vi "find_PipObject_by_InnerSwitchName.vi"(10 "inner switch name":string, 11 "PipObj Array in":refnum<class "Pipette.lvclass">[](array[class])) -> (0 "index of Object in Array":i32, 1 "found?":bool, 2 "found PipObj out":refnum<class "Pipette.lvclass">, 3 "PipObj Array out":refnum<class "Pipette.lvclass">[](array[class]))   [LabVIEW 2017]
doc: "Find the correct PipetteObject by the Name of the Inner Switch"
uses:
  Classes/Pipette/Pipette.lvclass
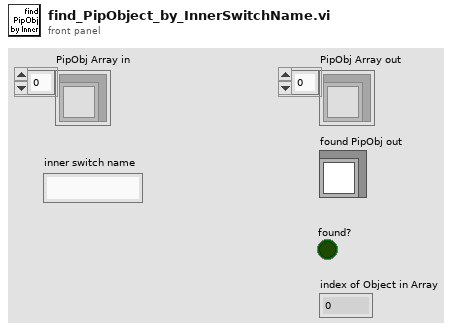
[diagram p1: front panel]
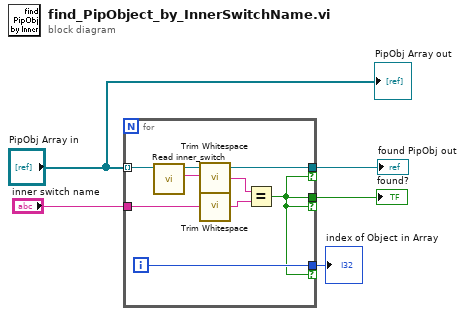
[diagram p0: block diagram]
diagram:
  n1 = for {
    tunnel: "inner switch name" -> [w13]
    tunnel: [w10] -> w4 if=w6
    tunnel: "PipObj Array in" -> [w8] mode=indexing
    tunnel: [w6] -> w3 if=w6
    tunnel: [w7] -> w1 if=w6
    i -> [w7]
    n2 = call-dynamic "Read inner_switch.vi"("Pipette in"=w8) -> ("inner_switch"=w9:string, "Pipette out"=w10:refnum<class "Pipette.lvclass">)  [unwired: 8 in, 1 out]
    n3 = call <vilib>:"Trim Whitespace.vi"("string"=w9) -> ("trimmed string"=w12:string)  [unwired: 1 in]
    n4 = call <vilib>:"Trim Whitespace.vi"("string"=w13) -> ("trimmed string"=w11:string)  [unwired: 1 in]
    n5 = Equal?(x=w12, y=w11) -> (x = y?=w6:bool)
  }
  "found PipObj out" <- w4
  "found?" <- w3
  "index of Object in Array" <- w1
  "PipObj Array out" <- "PipObj Array in"
